vi "Read configuration.vi"(8 "error in":errorcluster, 11 "fixed channel editor in":refnum<class "fixed channel editor.lvclass">) -> (0 "error out":errorcluster, 2 "configuration":refnum<class "NISE_CEF_serializable configuration.lvclass">, 3 "fixed channel editor out":refnum<class "fixed channel editor.lvclass">)   [LabVIEW 2013, in "fixed channel editor.lvclass"]
uses:
  fixed channel editor.lvclass
  <vilib>/NI/Configuration Framework/serializable configuration/NISE_CEF_serializable configuration.lvclass
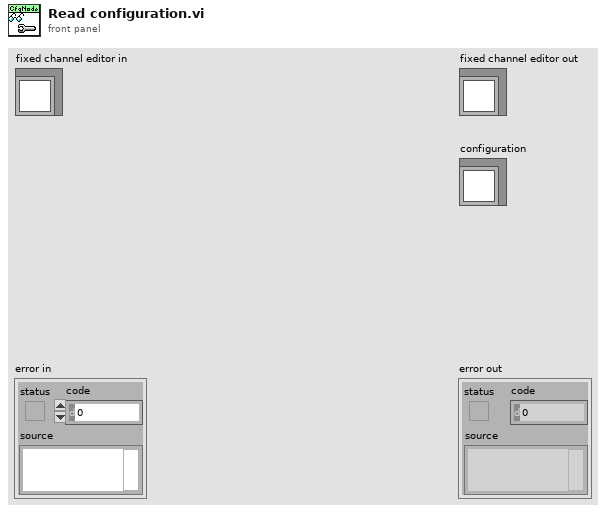
[diagram p1: front panel]
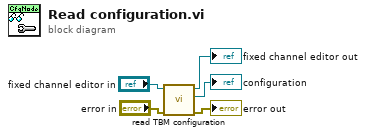
[diagram p0: block diagram]
diagram:
  n1 = call-dynamic "read TBM configuration.vi"("error in"="error in", "fixed module parent implementation editor node in"="fixed channel editor in") -> ("error out"=→"error out":errorcluster, "configuration"=→"configuration":refnum<class "TBM configuration.lvclass">, "fixed module parent implementation editor node out"=→"fixed channel editor out":refnum<class "fixed channel editor.lvclass">)  [unwired: 7 in]
